vi "Read Meas 34420.vi"(0 "address string":string, 1 "Software Trigger (F: OFF)":bool, 2 "Buffer (F: Internal)":bool, 3 "error in (no error)":errorcluster, 4 "Timeout (90000 ms)":u32=90000) -> (5 "Measurement":dbl[](array[numeric]) format="%.4e", 6 "error out":errorcluster {"code" format="%.0x"})   [LabVIEW 2014]
doc: "This VI will read whatever measurement has been selected from the measurement config or math config VI's. This includes dB, dBm, null, and limit.\n\nThe VI will wait up to the timeout value for data to become available. If the time expires prior to reading the data, you will receive a timeout error. The meaning of \"timeout\" is dependent upon the interface used and number of points collected. See below for details.\n\nGPIB\ninternal buffer (<512 points) -- RQS is asserted only after all data is collected and generally\n requires more time than VISA Read. Thus timeout is essentially the time needed for all\n data to be collected and RQS assented (VISA RQS timeout). \n\noutput buffer -- RQS is asserted after the first trigger point and then the driver waits on the\n meter to transmit data. Thus timeout is essentially the time needed for all data to be\n transmitted (VISA Read timeout).\n\n\nSerial (Not GPIB)\ninternal buffer (<512 points) -- Data transmission only begins after all data is collected and\n generally requires more time than VISA Read.\n\noutput buffer -- Data transmission begins immediately.\n\nIn both cases, the driver continually polls (ASRL Avail Num) the seral buffer and then reads only the data present. Although less efficient than performing a single VISA Read, this method significantly reduces processor overhead and frees system resources. Timeout is calculated using the tick count and is the time required for data collection and transmission. The VISA Read uses the default timeout value specified in HP34401A Initialize.vi. A VISA Read timeout is highly unlikely since data is being read from the seral buffer and not from the meter."
panel:
  # "ON\nOFF"
  # "Output\nInternal"
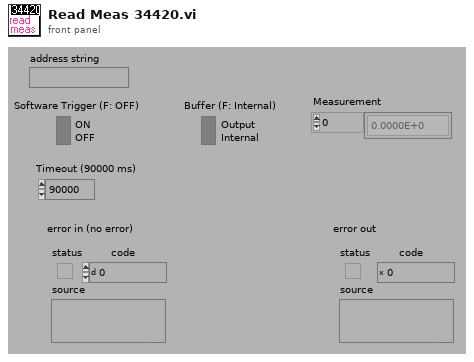
[diagram p1: front panel]
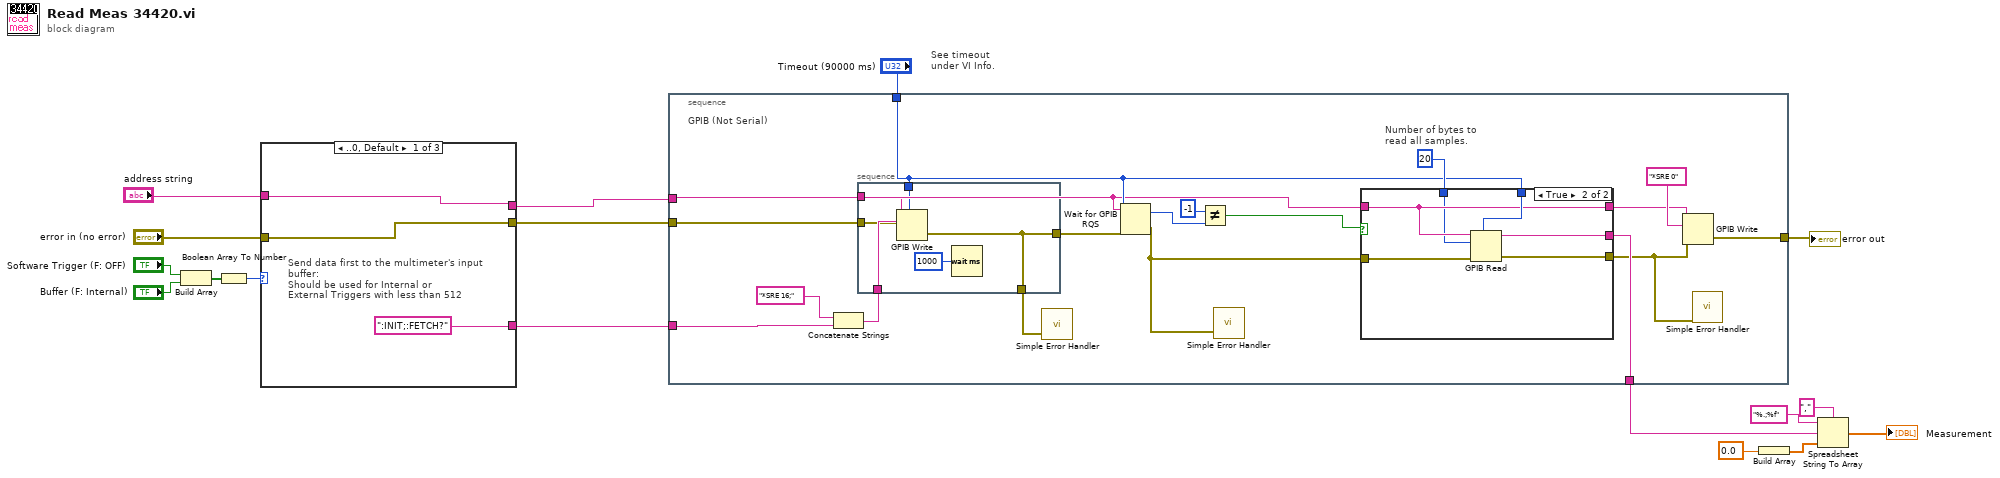
[diagram p0: block diagram]
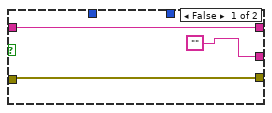
[diagram p2: hidden frame]
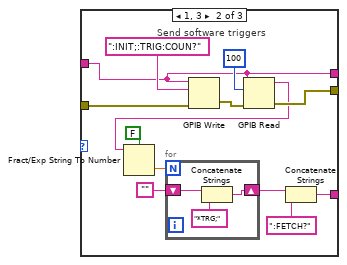
[diagram p3: hidden frame]
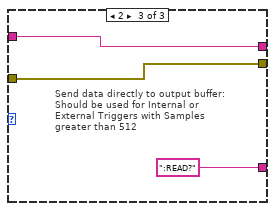
[diagram p4: hidden frame]
diagram:
  # "See timeout\nunder VI Info."
  n1 = Build Array("Software Trigger (F: OFF)", "Buffer (F: Internal)") -> (w15:bool[])
  n2 = Boolean Array To Number(Boolean array=w15) -> (number=w14:u32)
  n3 = case "Case" shown="..0, Default" w14 {
    tunnel: "error in (no error)" -> [w20 w28 w38]
    tunnel: [w20 w27 w38] -> w2
    tunnel: [":INIT;:FETCH?" w26 ":READ?"] -> w5
    tunnel: "address string" -> [w18 w21 w37]
    tunnel: [w18 w21 w37] -> w3
    frame ..0, Default {
      # "Send data first to the multimeter's input buffer:\nShould be used for Internal or \nExternal Triggers with less than 512"
    }
    frame 1, 3 {
      # "Send software triggers"
      n4 = GPIB Write(0:w21, 1:":INIT;:TRIG:COUN?", 3:w28) -> (6:w32:errorcluster)  [unwired: 2 in, 1 out]
      n5 = GPIB Read(0:w21, 1:u32 100, 3:w32) -> (5:w22:string, 7:w27:errorcluster)  [unwired: 2 in, 1 out]
      n6 = Fract/Exp String To Number(use system decimal point (T)=FALSE, string=w22) -> (number=w31:dbl)  [unwired: 2 in, 1 out]
      n7 = for {
        N: w31 -> [_]
        shift-right: [w35] -> w30
        shift-left: "" -> [w36]
        n8 = Concatenate Strings(w36, "*TRG;") -> (w35:string)
      }
      n9 = Concatenate Strings(w30, ":FETCH?") -> (w26:string)
    }
    frame 2 {
      # "Send data directly to output buffer:\nShould be used for Internal or \nExternal Triggers with Samples \ngreater than 512"
    }
  }
  n10 = stacked-sequence {
    tunnel: [w57] -> w1
    tunnel: [w52] -> w13
    tunnel: "Timeout (90000 ms)" -> [w45]
    tunnel: w5 -> [w54]
    tunnel: w3 -> [w44]
    tunnel: w2 -> [w50]
    frame #0 {
      # "Number of bytes to \nread all samples."
      # "GPIB (Not Serial)"
      n11 = Concatenate Strings("*SRE 16;", w54) -> (w51:string)
      n12 = stacked-sequence {
        tunnel: w51 -> [w63]
        tunnel: w50 -> [w62]
        tunnel: w45 -> [w61]
        tunnel: w44 -> [w59]
        tunnel: [w60] -> w47
        tunnel: [w60] -> w46
        frame #0 {
          n13 = GPIB Write(0:w59, 1:w63, 3:w62, 4:w61) -> (6:w60:errorcluster)  [unwired: 1 in, 1 out]
          n14 = Wait (ms)(milliseconds to wait=u32 1000) -> ()  [unwired: 1 out]
        }
      }
      n15 = call <vilib>:"Simple Error Handler.vi"("error in (no error)"=w47) -> ()  [unwired: 4 in, 5 out]
      n16 = Wait for GPIB RQS(2:w46, 3:w45, 4:w44) -> (0:w41:errorcluster, 1:w43:i16)
      n17 = Not Equal?(x=i16 -1, y=w43) -> (x != y?=w40:bool)
      n18 = call <vilib>:"Simple Error Handler.vi"("error in (no error)"=w41) -> ()  [unwired: 4 in, 5 out]
      n19 = case shown="True" w40 {
        tunnel: w45 -> [_ w72]
        tunnel: [w64 w71] -> w49
        tunnel: w44 -> [w66 w70]
        tunnel: [w66 w70] -> w53
        tunnel: ["" w69] -> w52
        tunnel: u32 20 -> [_ w68]
        tunnel: w41 -> [w64 w67]
        frame False {
        }
        frame True {
          n20 = GPIB Read(0:w70, 1:w68, 3:w67, 4:w72) -> (5:w69:string, 7:w71:errorcluster)  [unwired: 1 in, 1 out]
        }
      }
      n21 = GPIB Write(0:w53, 1:"*SRE 0", 3:w49) -> (6:w57:errorcluster)  [unwired: 2 in, 1 out]
      n22 = call <vilib>:"Simple Error Handler.vi"("error in (no error)"=w49) -> ()  [unwired: 4 in, 5 out]
    }
  }
  "error out" <- w1
  n23 = Build Array(0.0) -> (w8:dbl[])
  n24 = Spreadsheet String To Array(delimiter (Tab)=",", format string="%.;%f", spreadsheet string=w13, array type (2D Dbl)=w8) -> (array=→"Measurement":dbl[])
